vi "Train_GenerateVelocityofLeftRightWheels.vi"(11 "samples":i32=25) -> (3 "speed of Left and Right Wheels (rad/s)":cluster{dbl, dbl}[](array[cluster]))   [LabVIEW 2017]
uses:
  <vilib>/Analysis/1siggen.llb/Ramp Pattern by Delta.vi
  <vilib>/Analysis/NI_AALBase.lvlib
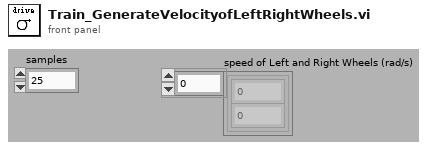
[diagram p1: front panel]
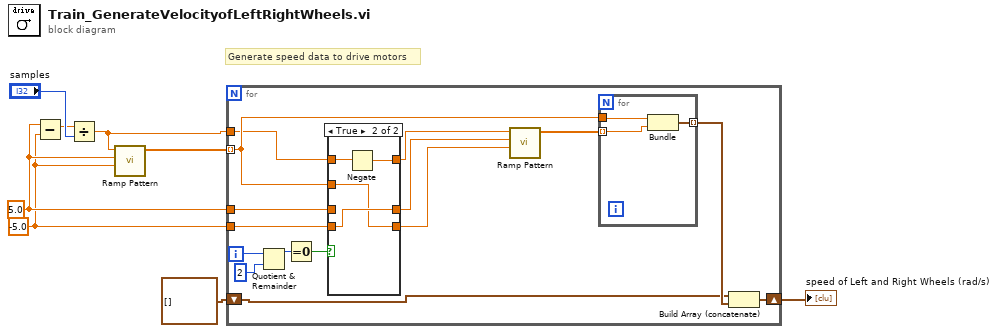
[diagram p0: block diagram]
diagram:
  w4 = -5.0 ("start")
  w5 = 5.0 ("end")
  # "Generate speed data to drive motors"
  n1 = Subtract(x=w5, y=w4) -> (x-y=w2:dbl)
  n2 = Divide(x=w2, y="samples") -> (x/y=w1:dbl)
  n3 = call-poly <vilib>:"Ramp Pattern.vi"("start"=w4, "end"=w5, "delta"=w1) -> ("Ramp Pattern"=w8:dbl[])  [unwired: 6 in, 2 out]
  n4 = for {
    tunnel: w8 -> [w11] mode=indexing
    tunnel: w5 -> [w19]
    tunnel: w4 -> [w18]
    tunnel: w1 -> [w10]
    shift-right: [w13] -> w6
    shift-left: cluster{dbl, dbl}[] [] -> [w12]
    i -> [w23]
    n5 = Quotient & Remainder(x=w23, y=2) -> (x-y*floor(x/y)=w21:i32)  [unwired: 1 out]
    n6 = Equal To 0?(x=w21) -> (x = 0?=w20:bool)
    n7 = case shown="True" w20 {
      tunnel: w19 -> [_ _]
      tunnel: w18 -> [w29 w33]
      tunnel: [w28 w33] -> w17
      tunnel: [w29 w32] -> w16
      tunnel: w11 -> [w28 w32]
      tunnel: w10 -> [w27 w31]
      tunnel: [w27 w30] -> w9
      frame False {
      }
      frame True {
        n8 = Negate(x=w31) -> (-x=w30:dbl)
      }
    }
    n9 = call-poly <vilib>:"Ramp Pattern.vi"("start"=w16, "end"=w17, "delta"=w9) -> ("Ramp Pattern"=w15:dbl[])  [unwired: 6 in, 2 out]
    n10 = for {
      tunnel: w15 -> [w25] mode=indexing
      tunnel: w11 -> [w26]
      tunnel: [w24] -> w14 mode=indexing
      n11 = Bundle(w26, w25) -> (w24:cluster{dbl, dbl})  [unwired: 1 in]
    }
    n12 = Build Array (concatenate)(w12, w14) -> (w13:cluster{dbl, dbl}[])
  }
  "speed of Left and Right Wheels (rad/s)" <- w6
